vi "Chirp-Compute Max Level.vi"(0 "Chirp Train":T3, 5 "Level in":T1, 9 "Sampling Rate (Hz)":dbl, 11 "error in (no error)":errorcluster) -> (4 "Numeric":dbl, 6 "Level out":T1, 15 "error out":errorcluster)   [LabVIEW 2020]
uses:
  Chirp Train.ctl
  Chirp Train Params.ctl
  Controls/Level XCtl/Level Data.ctl
  Controls/Level XCtl/Level Units.ctl
  <vilib>/Analysis/5stat.llb/RMS (DBL).vi
  PXI DAQ VIs/DAQ Engine VIs/PXI Globals.vi
  Utility VIs/Math VIs/Linear to dB (scalar).vi
  <vilib>/Analysis/NI_AALPro.lvlib
  Controls/Level XCtl/Level XCtl.xctl
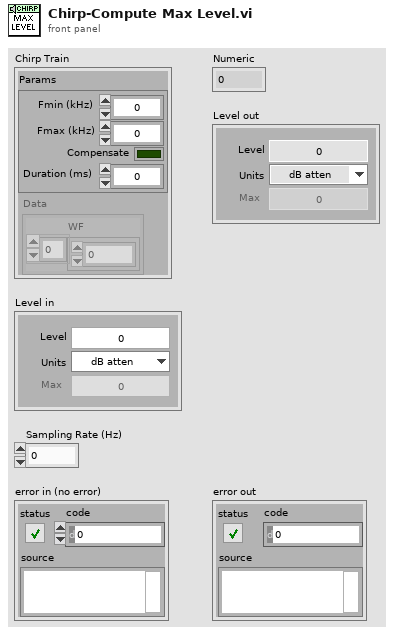
[diagram p1: front panel]
types:
  T1 = typedef "Level XCtl.xctl/Level Data.ctl" = cluster{"Level":dbl, "Units":T2, "Max":dbl, "Multiplier":dbl, "Cal File":path, "Cal":cluster{"Freq (Hz)":dbl[], "Mag (dB SPL)":dbl[], "Phase (deg)":dbl[]}}
  T2 = typedef "Level Units.ctl" = enum16{"dB atten", "dB SPL", "dB re 1 Vrms", "dB V/Hz½", "mW", "dB HL", "Volts", "dB mW"}
  T3 = typedef "Chirp Train.ctl" = cluster{"Params":T4, "Data":cluster{"WF":dbl[]}}
  T4 = typedef "Chirp Train Params.ctl" = cluster{"Fmin (kHz)":dbl, "Fmax (kHz)":dbl, "Compensate":bool, "Duration (ms)":dbl}
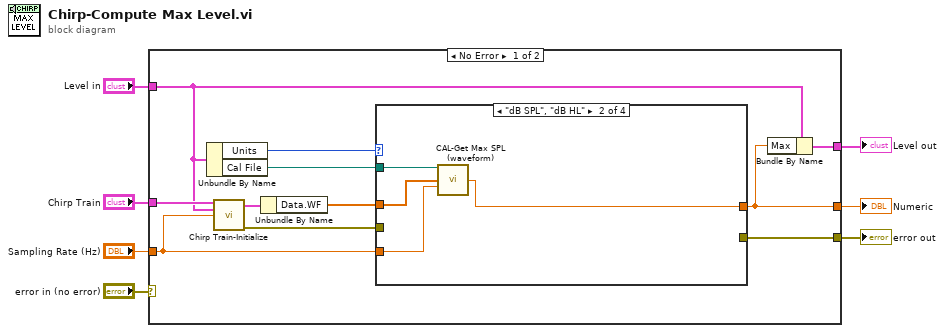
[diagram p0: block diagram]
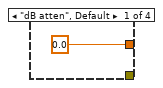
[diagram p2: hidden frame]
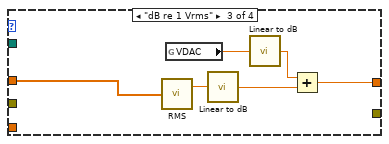
[diagram p3: hidden frame]
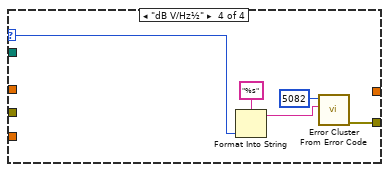
[diagram p4: hidden frame]
diagram:
  n1 = case shown="No Error" "error in (no error)" {
    selector: "error in (no error)" -> [_ w35]
    tunnel: [w8 w35] -> w2
    tunnel: [w14 _] -> w3
    tunnel: [w13 _] -> w4
    tunnel: "Level in" -> [w15 _]
    tunnel: "Chirp Train" -> [w16 _]
    tunnel: "Sampling Rate (Hz)" -> [w12 _]
    frame No Error {
      n2 = Unbundle By Name(w15) -> ("Units"=w18:T2, "Cal File"=w17:path)
      n3 = call "Chirp Train-Initialize.vi"("Chirp Train in"=w16, "Level"=w15, "Sampling rate (Hz)"=w12) -> ("Chirp Train out"=w11:T3, "error out"=w9:errorcluster)  [unwired: 11 in]
      n4 = Unbundle By Name(w11) -> ("Data.WF"=w10:dbl[])
      n5 = case shown="\"dB SPL\", \"dB HL\"" w18 {
        selector: w18 -> [_ _ _ w30]
        tunnel: w12 -> [_ w21 _ _]
        tunnel: [0.0 ("Reference Level") w20 w28 _] -> w14
        tunnel: w17 -> [_ w23 _ _]
        tunnel: w10 -> [_ w22 w24 _]
        tunnel: w9 -> [_ _ _ _]
        tunnel: [_ _ _ w31] -> w8
        frame "dB atten", Default {
        }
        frame "dB SPL", "dB HL" {
          n6 = call "CAL-Get Max SPL (waveform).vi"("Cal File"=w23, "Y"=w22, "Sampling Rate (Hz)"=w21) -> ("Max SPL"=w20:dbl)  [unwired: 11 in, 1 out]
        }
        frame "dB re 1 Vrms" {
          n7 = call-poly <vilib>:"RMS.vi"("X"=w24) -> ("rms value"=w26:dbl)  [unwired: 1 out]
          n8 = global read "PXI Globals.vi" "VDAC"() -> (w29:dbl)
          n9 = call-poly "Linear to dB.vi"("Linear"=w26) -> ("dB"=w25:dbl)
          n10 = call-poly "Linear to dB.vi"("Linear"=w29) -> ("dB"=w27:dbl)
          n11 = Add(x=w27, y=w25) -> (x+y=w28:dbl)
        }
        frame "dB V/Hz½" {
          n12 = Format Into String(format string="%s", w30) -> (resulting string=w33:string)  [unwired: 2 in, 1 out]
          n13 = call <vilib>:"Error Cluster From Error Code.vi"("error message (\"\")"=w33, "error code (0)"=5082) -> ("error out"=w31:errorcluster)  [unwired: 7 in]
        }
      }
      n14 = Bundle By Name(cluster=w15, "Max"=w14) -> (w13:T1)
    }
    frame Error {
    }
  }
  "Level out" <- w4
  "Numeric" <- w3
  "error out" <- w2
